vi "BRig_FPGA_v3,95.vi"() -> ()   [LabVIEW 2014]
uses:
  <vilib>/rvi/Emulation/niFpgaGetClockAttributes.vi
  <vilib>/rvi/Emulation/niFpgaSctlEmulationGetInTimedLoop.vi
  <vilib>/rvi/Emulation/niFpgaEmulationReportErrorSimple.vi
  <vilib>/rvi/eio/common/nirviEmuTemplateMethod_errors.vi
  <vilib>/rvi/Emulation/niFpgaCriticalErrorInLSC.vi
  <vilib>/eio/EIONode/EIONode.xnode
panel:
  out "AnaIn_1_0":u16
  out "AnaIn_1_1":u16
  out "AnaIn_1_2":u16
  out "AnaIn_1_3":u16
  out "AnaIn_1_4":u16
  out "AnaIn_0_4":u16
  out "AnaIn_0_3":u16
  out "AnaIn_0_2":u16
  out "AnaIn_0_1":u16
  out "AnaIn_0_0":u16
  in  "AI_newCycleFlag":bool
  in  "AnaOut1_Pair":u16
  in  "AnaOut0_Pair":u16
  out "fpga_solenoid_R":bool
  out "fpga_solenoid_L":bool
  out "fpga_laser2":bool
  out "fpga_laser1":bool
  in  "L2Led_ON":bool
  in  "L1Led_ON":bool
  in  "Rising(F)_or_Falling(T)":bool
  in  "Solenoid_trig_R":bool
  in  "Solenoid_trig_L":bool
  in  "Solenoid_nTotal_R":u32=100
  in  "Solenoid_nTotal_L":u32=100
  in  "L2Led_Baseline":bool
  in  "L1Led_Baseline":bool
  in  "CueLed_Baseline":bool
  in  "I_allReward":bool
  in  "AnaOut_1":u16
  in  "CueLed_Event":bool
  in  "CueLed_nValley":u32=100
  in  "CueLed_nPeak":u32=100
  in  "LC_Event_l2":bool
  in  "LC_Laser_l2":bool
  in  "LC_nShutter_l2":u32=100
  in  "LC_nValley_l2":u32=100
  in  "LC_nPeak_l2":u32=100
  in  "LR_wrong_nDelay_l2":u32
  in  "LR_reward_nDelay_l2":u32
  in  "LR_wrong_nTotal_l2":u32=100
  in  "LR_reward_nTotal_l2":u32=100
  in  "LR_wrong_laser_l2":bool
  in  "LR_wrong_Event_l2":bool
  in  "LR_reward_Laser_l2":bool
  in  "LR_reward_Event_l2":bool
  out "AnaIn_1":u16
  out "AnaIn_0":u16
  out "timeTrial_count":u32
  in  "timeTrial_trig":bool
  in  "k1__counter_per_ms":u16=100 min=100 max=40000 step=1
  in  "LC_nShutter_l1":u32=100
  in  "AnaOut_0":u16
  in  "LC_nValley_l1":u32=100
  in  "LC_nPeak_l1":u32=100
  in  "LC_Event_l1":bool
  in  "LR_wrong_nTotal_l1":u32=100
  in  "LR_wrong_nDelay_l1":u32
  in  "LR_reward_nTotal_l1":u32=100
  in  "LR_reward_nDelay_l1":u32
  in  "LR_reward_Event_l1":bool
  in  "LR_wrong_Event_l1":bool
  out "SelectWrong":bool
  out "SelectReward":bool
  in  "LR_wrong_Laser_l1":bool
  in  "LR_reward_Laser_l1":bool
  in  "Left(F)_or_Right(T)":bool
  in  "ignoreWrong":bool
  in  "SelectionState":bool
  in  "LC_Laser_l1":bool
  in  "FPGA_Stop":bool
  in  "audioTrigger_L":bool
  in  "audioTrigger_R":bool
  in  "audioFreq_L_kHz":u8=14 min=1 max=14 step=1
  in  "audioAmp_L":u16=1 min=1 max=32767 step=1
  in  "audioFreq_R_kHz":u8=14 min=1 max=14 step=1
  in  "audioAmp_R":u16=1 min=1 max=32767 step=1
  in  "A3_SL":bool
  in  "A1_SR":bool
  in  "Counts_Reset":bool
  out "A4_LickR":u32
  out "A2_LickL":u32
  in  "A6_Act":bool
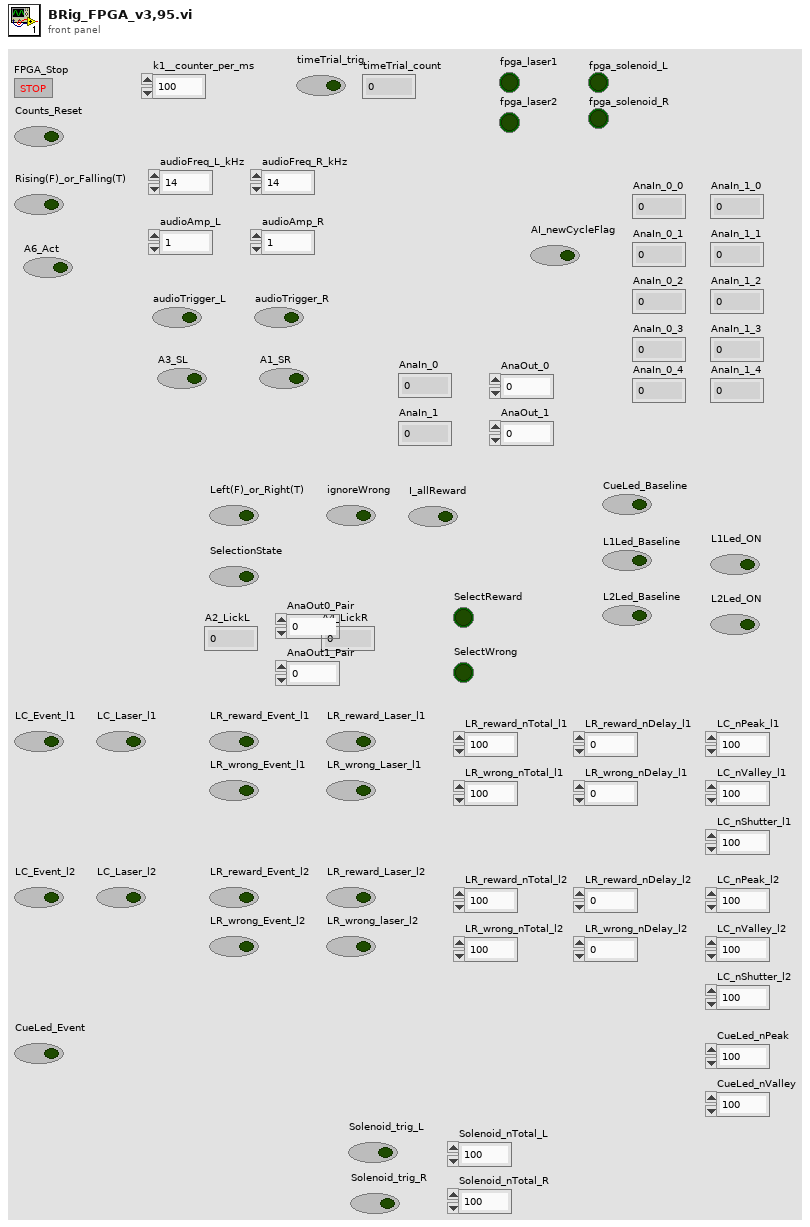
[diagram p1: front panel]
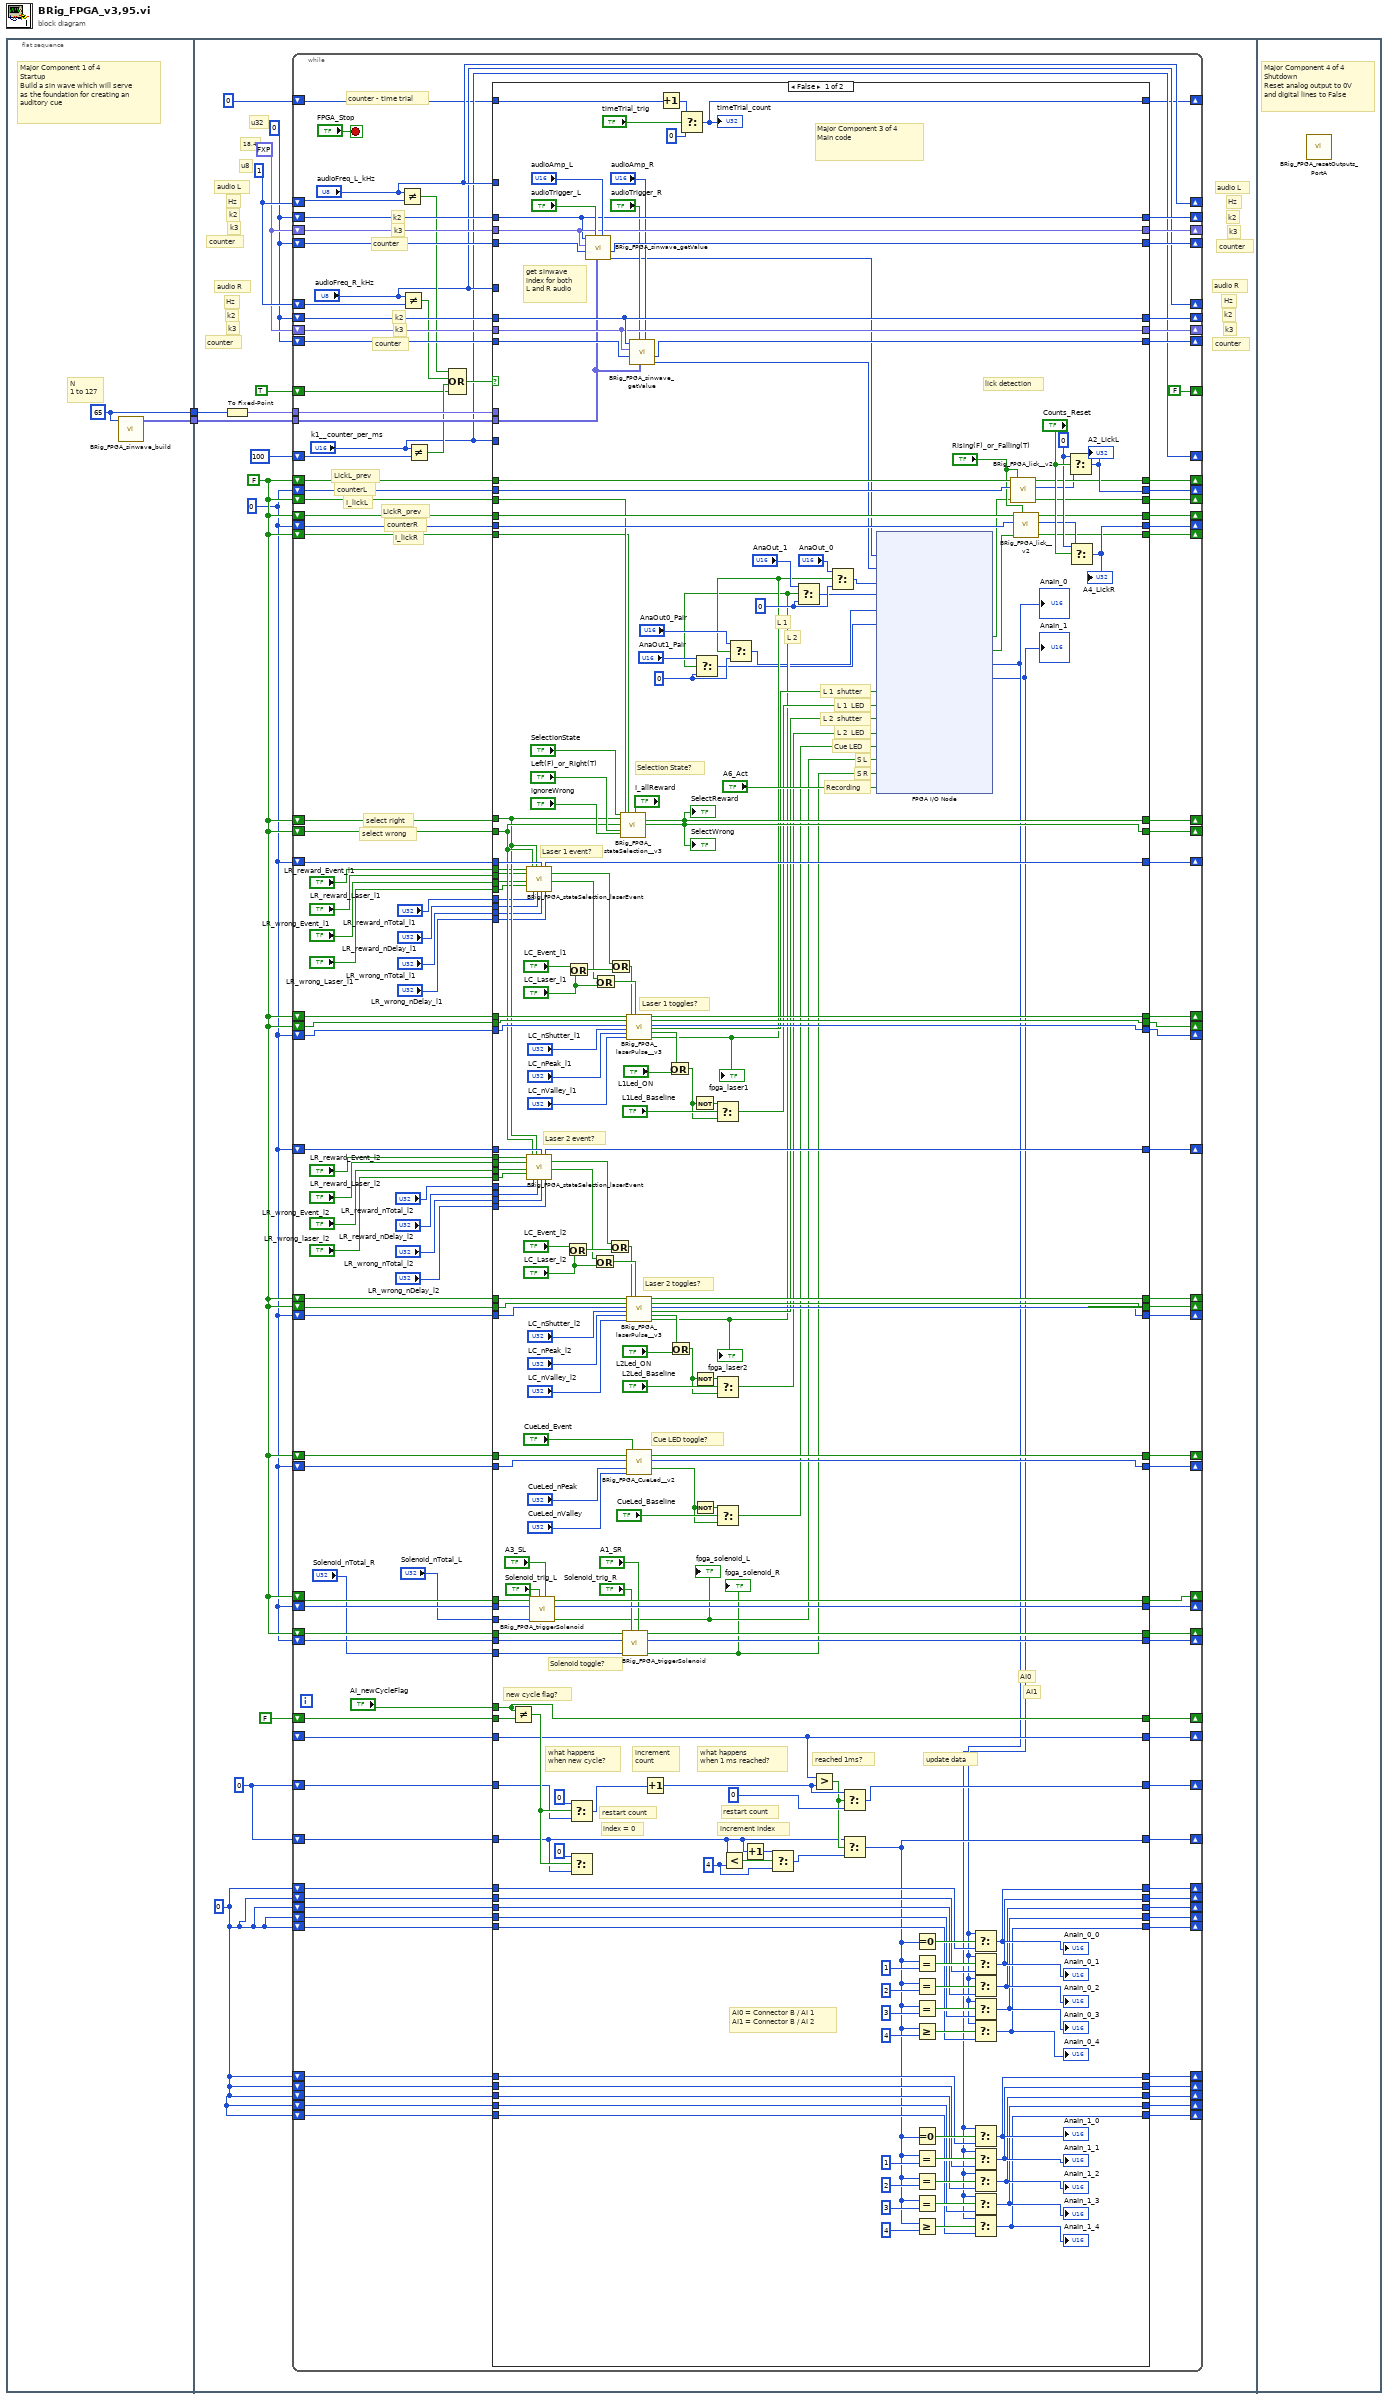
[diagram p0: block diagram]
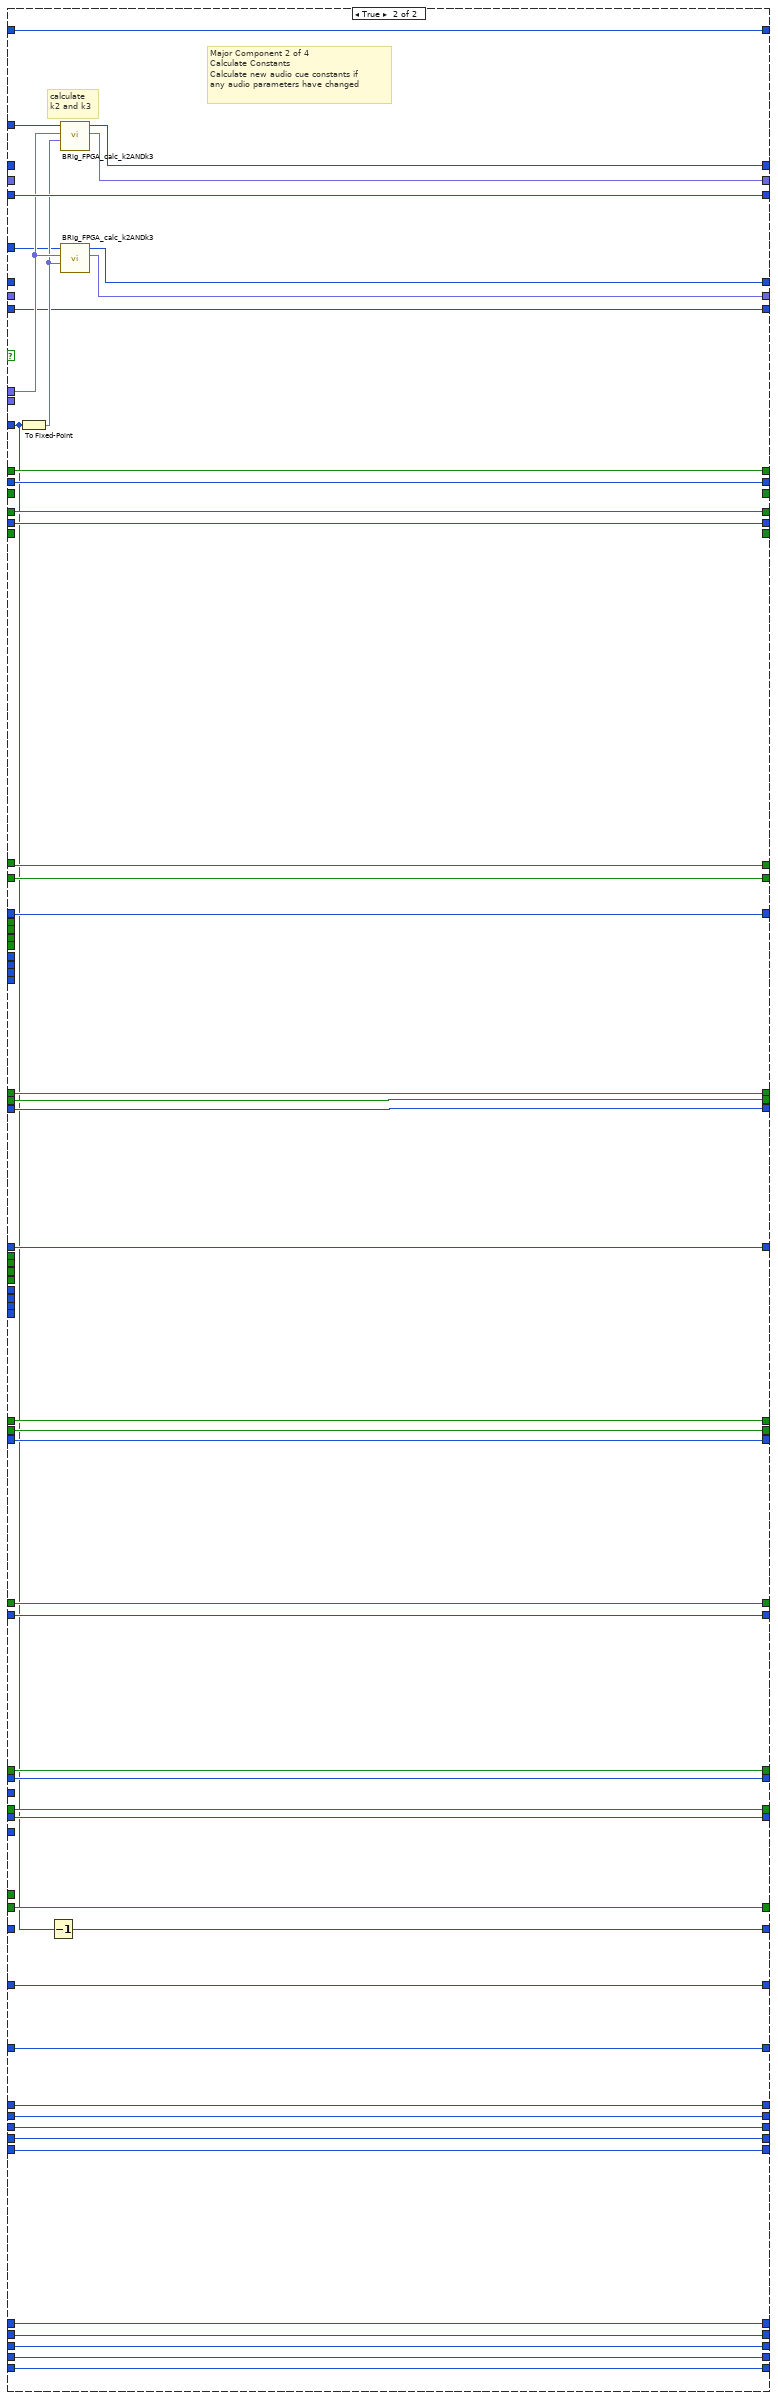
[diagram p2: hidden frame]
diagram:
  n1 = flat-sequence {
    tunnel: [w4] -> w2
    tunnel: [w3] -> w1
    tunnel: w2 -> [w18]
    tunnel: w1 -> [w17]
    frame #0 {
      w3 = 65 ("dimension size")
      # "Major Component 1 of 4\nStartup\nBuild a sin wave which will serve\nas the foundation for creating an\nauditory cue"
      # "N\n1 to 127"
      n2 = call "BRig_FPGA_sinwave_build.vi"("input_Npts"=w3) -> ("output_array_sin"=w4:fxp<+/-,16,2>[])  [unwired: 10 in]
    }
    frame #1 {
      w6 = u16 0
      w5 = u16 0
      w8 = u32 0
      w9 = FALSE
      w13 = u32 0
      w14 = fxp<+,18,4> 0.0
      w15 = u8 1
      # "counter"
      # "k3"
      # "k2"
      # "counter"
      # "k3"
      # "k2"
      # "counter"
      # "counter"
      # "u32"
      # "k3"
      # "k2"
      # "k3"
      # "18,4"
      # "u8"
      # "Hz"
      # "Hz"
      # "audio R"
      # "audio L"
      # "Hz"
      # "k2"
      # "Hz"
      # "audio R"
      # "audio L"
      n3 = To Fixed-Point(number=w17) -> (fixed-point=w16:fxp<+,7,7>)  [unwired: 1 in]
      n4 = while {
        shift-right: ["audioFreq_L_kHz"] -> _
        shift-left: w15 -> [w138]
        shift-right: [w132] -> _
        shift-left: w13 -> [w136]
        shift-right: ["audioFreq_R_kHz"] -> _
        shift-left: w15 -> [w128]
        tunnel: w18 -> [w135]
        tunnel: w16 -> [w134]
        shift-right: [w131] -> _
        shift-left: w14 -> [w133]
        shift-right: [w129] -> _
        shift-left: w13 -> [w130]
        shift-right: [w126] -> _
        shift-left: w13 -> [w127]
        shift-right: [w124] -> _
        shift-left: w14 -> [w125]
        shift-right: [w122] -> _
        shift-left: w13 -> [w123]
        shift-right: ["k1__counter_per_ms"] -> _
        shift-left: u16 100 ("y") -> [w121]
        shift-right: [FALSE] -> _
        shift-left: TRUE -> [w116]
        shift-right: [w109] -> _
        shift-left: w9 -> [w111]
        shift-right: [w108] -> _
        shift-left: w9 -> [w110]
        shift-right: [w106] -> _
        shift-left: w8 -> [w107]
        shift-right: [w104] -> _
        shift-left: w8 -> [w105]
        shift-right: [w101] -> _
        shift-left: w9 -> [w103]
        shift-right: [w100] -> _
        shift-left: w9 -> [w102]
        shift-right: [w98] -> _
        shift-left: w9 -> [w99]
        shift-right: [w96] -> _
        shift-left: w9 -> [w97]
        shift-right: [w94] -> _
        shift-left: u32 0 -> [w95]
        shift-right: [w92] -> _
        shift-left: w8 -> [w93]
        shift-right: [w91] -> _
        shift-left: w9 -> [w88]
        shift-right: [w90] -> _
        shift-left: w9 -> [w87]
        shift-right: [w89] -> _
        shift-left: w8 -> [w86]
        shift-right: [w84] -> _
        shift-left: w8 -> [w85]
        shift-right: [w83] -> _
        shift-left: w9 -> [w80]
        shift-right: [w82] -> _
        shift-left: w9 -> [w79]
        shift-right: [w81] -> _
        shift-left: w8 -> [w78]
        shift-right: [w77] -> _
        shift-left: w9 -> [w75]
        shift-right: [w76] -> _
        shift-left: w8 -> [w74]
        shift-right: [w56] -> _
        shift-left: w8 -> [w57]
        shift-right: [w53] -> _
        shift-left: w9 -> [w55]
        shift-right: [w50] -> _
        shift-left: w9 -> [w52]
        shift-right: [w49] -> _
        shift-left: w8 -> [w51]
        shift-right: [w33] -> _
        shift-left: FALSE -> [w46]
        shift-right: [w32] -> _
        shift-left: w6 -> [w44]
        shift-right: [w31] -> _
        shift-left: w6 -> [w43]
        shift-right: [w30] -> _
        shift-left: w5 -> [w45]
        shift-right: [w29] -> _
        shift-left: w5 -> [w41]
        shift-right: [w28] -> _
        shift-left: w5 -> [w40]
        shift-right: [w27] -> _
        shift-left: w5 -> [w39]
        shift-right: [w26] -> _
        shift-left: w5 -> [w42]
        shift-right: [w25] -> _
        shift-left: w5 -> [w38]
        shift-right: [w24] -> _
        shift-left: w5 -> [w37]
        shift-right: [w23] -> _
        shift-left: w5 -> [w36]
        shift-right: [w22] -> _
        shift-left: w5 -> [w35]
        shift-right: [w21] -> _
        shift-left: w5 -> [w34]
        shift-right: [w20] -> _
        shift-left: _ -> [w19]
        stop <- "FPGA_Stop" stop-if-true
        # "counter"
        # "k3"
        # "k2"
        # "counter"
        # "k3"
        # "k2"
        # "counter - time trial"
        # "I_lickR"
        # "counterR"
        # "LickR_prev"
        # "I_lickL"
        # "counterL"
        # "LickL_prev"
        # "select wrong"
        # "select right"
        n5 = Not Equal?(x="audioFreq_L_kHz", y=w138) -> (x != y?=w120:bool)
        n6 = Not Equal?(x="audioFreq_R_kHz", y=w128) -> (x != y?=w119:bool)
        n7 = Not Equal?(x="k1__counter_per_ms", y=w121) -> (x != y?=w117:bool)
        n8 = Compound Arithmetic op=OR(w120, w119, w117, w116) -> (w118:bool)
        n9 = case shown="False" w118 {
          tunnel: w136 -> [w334 _]
          tunnel: "audioFreq_L_kHz" -> [_ w395]
          tunnel: w135 -> [w327 _]
          tunnel: w134 -> [_ w391]
          tunnel: "k1__counter_per_ms" -> [_ w352]
          tunnel: w133 -> [w335 _]
          tunnel: [w334 w394] -> w132
          tunnel: [w335 w393] -> w131
          tunnel: w130 -> [w339 w392]
          tunnel: [w336 w392] -> w129
          tunnel: w127 -> [w331 _]
          tunnel: [w331 w387] -> w126
          tunnel: w125 -> [w330 _]
          tunnel: [w330 w388] -> w124
          tunnel: w123 -> [w333 w386]
          tunnel: "audioFreq_R_kHz" -> [_ w389]
          tunnel: [w332 w386] -> w122
          tunnel: w111 -> [w322 w385]
          tunnel: w110 -> [w321 w384]
          tunnel: [w326 w385] -> w109
          tunnel: [w319 w384] -> w108
          tunnel: w107 -> [w323 w383]
          tunnel: [w349 w383] -> w106
          tunnel: w105 -> [w320 w382]
          tunnel: [w346 w382] -> w104
          tunnel: w103 -> [w277 w381]
          tunnel: w102 -> [w278 w380]
          tunnel: [w297 w381] -> w101
          tunnel: [w342 w380] -> w100
          tunnel: [w312 w377] -> w91
          tunnel: [w313 w376] -> w90
          tunnel: [w314 w375] -> w89
          tunnel: w99 -> [w316 _]
          tunnel: [w325 _] -> w98
          tunnel: w97 -> [w315 _]
          tunnel: [w317 _] -> w96
          tunnel: w95 -> [w304 w379]
          tunnel: [w301 w379] -> w94
          tunnel: w93 -> [w296 w378]
          tunnel: [w295 w378] -> w92
          tunnel: w88 -> [w294 w377]
          tunnel: w87 -> [w293 w376]
          tunnel: w86 -> [w292 w375]
          tunnel: w85 -> [w280 w374]
          tunnel: [w279 w374] -> w84
          tunnel: [w275 w373] -> w83
          tunnel: [w274 w372] -> w82
          tunnel: [w273 w371] -> w81
          tunnel: w80 -> [w272 w373]
          tunnel: w79 -> [w271 w372]
          tunnel: w78 -> [w270 w371]
          tunnel: [w267 w370] -> w77
          tunnel: [w266 w369] -> w76
          tunnel: w75 -> [w265 w370]
          tunnel: w74 -> [w264 w369]
          tunnel: "LR_reward_Event_l1" -> [w250 _]
          tunnel: "LR_reward_Laser_l1" -> [w249 _]
          tunnel: "LR_wrong_Event_l1" -> [w248 _]
          tunnel: "LR_wrong_Laser_l1" -> [w247 _]
          tunnel: "LR_reward_nTotal_l1" -> [w246 _]
          tunnel: "LR_reward_nDelay_l1" -> [w245 _]
          tunnel: "LR_wrong_nTotal_l1" -> [w244 _]
          tunnel: "LR_wrong_nDelay_l1" -> [w243 _]
          tunnel: "LR_reward_Event_l2" -> [w242 _]
          tunnel: "LR_reward_Laser_l2" -> [w241 _]
          tunnel: "LR_wrong_Event_l2" -> [w240 _]
          tunnel: "LR_wrong_laser_l2" -> [w239 _]
          tunnel: "LR_reward_nTotal_l2" -> [w238 _]
          tunnel: "LR_reward_nDelay_l2" -> [w237 _]
          tunnel: "LR_wrong_nTotal_l2" -> [w236 _]
          tunnel: "LR_wrong_nDelay_l2" -> [w235 _]
          tunnel: w57 -> [w234 w368]
          tunnel: [w229 w368] -> w56
          tunnel: w55 -> [w233 w367]
          tunnel: "Solenoid_nTotal_L" -> [w232 _]
          tunnel: [w228 w367] -> w53
          tunnel: w52 -> [w225 w366]
          tunnel: w51 -> [w224 w365]
          tunnel: [w223 w366] -> w50
          tunnel: [w222 w365] -> w49
          tunnel: "Solenoid_nTotal_R" -> [w221 _]
          tunnel: "AI_newCycleFlag" -> [w154 _]
          tunnel: w46 -> [w167 w364]
          tunnel: w45 -> [w166 w362]
          tunnel: w44 -> [w165 w351]
          tunnel: w43 -> [w164 w363]
          tunnel: w42 -> [w163 w358]
          tunnel: w41 -> [w162 w361]
          tunnel: w40 -> [w161 w360]
          tunnel: w39 -> [w160 w359]
          tunnel: w38 -> [w159 w357]
          tunnel: w37 -> [w158 w356]
          tunnel: w36 -> [w157 w355]
          tunnel: w35 -> [w156 w354]
          tunnel: w34 -> [w155 w353]
          tunnel: [w154 w364] -> w33
          tunnel: [w152 w351] -> w32
          tunnel: [w151 w363] -> w31
          tunnel: [w148 w362] -> w30
          tunnel: [w147 w361] -> w29
          tunnel: [w146 w360] -> w28
          tunnel: [w145 w359] -> w27
          tunnel: [w144 w358] -> w26
          tunnel: [w143 w357] -> w25
          tunnel: [w142 w356] -> w24
          tunnel: [w141 w355] -> w23
          tunnel: [w140 w354] -> w22
          tunnel: [w139 w353] -> w21
          tunnel: w19 -> [w153 _]
          tunnel: [w153 w350] -> w20
          frame False {
            w186 = u16 4 ("y")
            w202 = u16 0 ("f")
            w261 = u16 0 ("f")
            w347 = u32 0 ("t")
            # "AI0 = Connector B / AI 1\nAI1 = Connector B / AI 2"
            # "increment index"
            # "restart count"
            # "index = 0"
            # "restart count"
            # "AI1"
            # "AI0"
            # "update data"
            # "reached 1ms?"
            # "increment\ncount"
            # "what happens\nwhen new cycle?"
            # "what happens\nwhen 1 ms reached?"
            # "new cycle flag?"
            # "Cue LED"
            # "L 2  shutter"
            # "L 2  LED"
            # "L 1  shutter"
            # "L 1  LED"
            # "Recording"
            # "S L"
            # "S R"
            # "L 2"
            # "L 1"
            # "Solenoid toggle?"
            # "Cue LED toggle?"
            # "Laser 2 toggles?"
            # "Laser 2 event?"
            # "Laser 1 toggles?"
            # "Selection State?"
            # "Laser 1 event?"
            # "Major Component 3 of 4\nMain code"
            # "get sinwave\nindex for both\nL and R audio"
            # "lick detection"
            n10 = Not Equal?(x=w154, y=w167) -> (x != y?=w192:bool)
            n11 = call "BRig_FPGA_stateSelection_laserEvent.vi"("I_LR_reward"=w250, "I_LR_reward_laser"=w249, "I_LR_wrong"=w248, "I_LR_wrong_laser"=w247, "I_selectWrong"=w278, "laser_reward_nTotal"=w246, "I_selectReward"=w277, "laser_reward_nDelay"=w245, "counter"=w296, "laser_wrong_nTotal"=w244, "laser_wrong_nDelay"=w243) -> ("output_counter"=w295:u32, "output_I_laserEvent"=w291:bool, "output_I_laserOn"=w290:bool)  [unwired: 6 in]
            n12 = call "BRig_FPGA_stateSelection_laserEvent.vi"("I_LR_reward"=w242, "I_LR_reward_laser"=w241, "I_LR_wrong"=w240, "I_LR_wrong_laser"=w239, "I_selectWrong"=w278, "laser_reward_nTotal"=w238, "I_selectReward"=w277, "laser_reward_nDelay"=w237, "counter"=w280, "laser_wrong_nTotal"=w236, "laser_wrong_nDelay"=w235) -> ("output_counter"=w279:u32, "output_I_laserEvent"=w276:bool, "output_I_laserOn"=w281:bool)  [unwired: 6 in]
            n13 = call "BRig_FPGA_triggerSolenoid.vi"("input_Solenoid_MTrig"="A3_SL", "input_Solenoid_trig"="Solenoid_trig_L", "input_threshold"=w232, "input_counter"=w234, "input_trig"=w233) -> ("output_Solenoid_OnOff"=w205:bool, "output_counter"=w229:u32, "output_trig"=w228:bool)  [unwired: 4 in]
            "fpga_solenoid_L" <- w205
            n14 = Or(x="LC_Event_l2", y="LC_Laser_l2") -> (x .or. y?=w285:bool)
            n15 = Or(x="LC_Event_l1", y="LC_Laser_l1") -> (x .or. y?=w308:bool)
            n16 = Select(t=u16 0, s=w192, f=w165) -> (s? t:f=w191:u16)
            n17 = Select(t=u16 0 ("f"), s=w192, f=w164) -> ()  [unwired: 1 out]
            n18 = call "BRig_FPGA_sinwave_getValue.vi"("audioAmp"="audioAmp_L", "sinwave"=w327, "audioTrigger"="audioTrigger_L", "counter"=w339, "k3"=w335, "k2"=w334) -> ("output_audioValue"=w299:i16, "output_counter"=w336:u32)  [unwired: 4 in]
            n19 = Or(x=w281, y="LC_Laser_l2") -> (x .or. y?=w283:bool)
            n20 = Or(x=w290, y="LC_Laser_l1") -> (x .or. y?=w306:bool)
            n21 = Or(x=w276, y=w285) -> (x .or. y?=w282:bool)
            n22 = Or(x=w291, y=w308) -> (x .or. y?=w305:bool)
            n23 = call "BRig_FPGA_stateSelection__v3.vi"("I_selectionState"="SelectionState", "I_selectRight"=w277, "I_selectWrong"=w278, "I_Left(F)_or_Right(T)"="Left(F)_or_Right(T)", "I_ignoreWrong"="ignoreWrong", "I_lickL"=w316, "I_lickR"=w315, "I_allReward"="I_allReward") -> ("output__I_selectRight"=w297:bool, "output__I_selectWrong"=w342:bool)  [unwired: 18 in]
            "SelectWrong" <- w342
            "SelectReward" <- w297
            n24 = call "BRig_FPGA_triggerSolenoid.vi"("input_Solenoid_MTrig"="A1_SR", "input_Solenoid_trig"="Solenoid_trig_R", "input_threshold"=w221, "input_counter"=w224, "input_trig"=w225) -> ("output_Solenoid_OnOff"=w204:bool, "output_counter"=w222:u32, "output_trig"=w223:bool)  [unwired: 4 in]
            "fpga_solenoid_R" <- w204
            n25 = call "BRig_FPGA_laserPulse__v3.vi"("I_shutter"=w294, "I_peak"=w293, "count"=w292, "laser_Nshutter"="LC_nShutter_l1", "laser_Npeak"="LC_nPeak_l1", "laser_Nvalley"="LC_nValley_l1", "I_laserEvent"=w305, "I_laser"=w306) -> ("output_I_shutter"=w312:bool, "output_I_peak"=w313:bool, "output_count"=w314:u32, "output_shutter"=w210:bool, "output_led"=w218:bool, "output_laser"=w200:bool)  [unwired: 6 in]
            "fpga_laser1" <- w200
            n26 = call "BRig_FPGA_laserPulse__v3.vi"("I_shutter"=w272, "I_peak"=w271, "count"=w270, "laser_Nshutter"="LC_nShutter_l2", "laser_Npeak"="LC_nPeak_l2", "laser_Nvalley"="LC_nValley_l2", "I_laserEvent"=w282, "I_laser"=w283) -> ("output_I_shutter"=w275:bool, "output_I_peak"=w274:bool, "output_count"=w273:u32, "output_shutter"=w208:bool, "output_led"=w215:bool, "output_laser"=w199:bool)  [unwired: 6 in]
            "fpga_laser2" <- w199
            n27 = call "BRig_FPGA_CueLed__v2.vi"("I_peak"=w265, "count"=w264, "laser_Npeak"="CueLed_nPeak", "laser_Nvalley"="CueLed_nValley", "I_CueLed_Event"="CueLed_Event") -> ("output_I_peak"=w267:bool, "output_count"=w266:u32, "output_led"=w255:bool)  [unwired: 12 in]
            n28 = call "BRig_FPGA_sinwave_getValue.vi"("audioAmp"="audioAmp_R", "sinwave"=w327, "audioTrigger"="audioTrigger_R", "counter"=w333, "k3"=w330, "k2"=w331) -> ("output_audioValue"=w298:i16, "output_counter"=w332:u32)  [unwired: 4 in]
            n29 = Increment(x=w191) -> (x+1=w190:u16)
            n30 = Increment(x=w304) -> (x+1=w303:u32)
            n31 = Or(x=w218, y="L1Led_ON") -> (x .or. y?=w217:bool)
            n32 = Or(x=w215, y="L2Led_ON") -> (x .or. y?=w214:bool)
            n33 = Select(t=w303, s="timeTrial_trig", f=u32 0) -> (s? t:f=w301:u32)
            "timeTrial_count" <- w301
            n34 = Not(x=w217) -> (.not. x?=w254:bool)
            n35 = Not(x=w214) -> (.not. x?=w252:bool)
            n36 = Not(x=w255) -> (.not. x?=w257:bool)
            n37 = Select(t="AnaOut1_Pair", s=w199, f=w202) -> (s? t:f=w198:u16)
            n38 = Select(t=w254, s="L1Led_Baseline", f=w217) -> (s? t:f=w209:bool)
            n39 = Select(t=w252, s="L2Led_Baseline", f=w214) -> (s? t:f=w207:bool)
            n40 = Select(t=w257, s="CueLed_Baseline", f=w255) -> (s? t:f=w206:bool)
            n41 = Less?(x=w164, y=w186) -> (x < y?=w196:bool)
            n42 = Select(t="AnaOut0_Pair", s=w200, f=w202) -> (s? t:f=w197:u16)
            n43 = Increment(x=w164) -> (x+1=w195:u16)
            n44 = Select(t=w195, s=w196, f=w186) -> (s? t:f=w187:u16)
            n45 = Select(t="AnaOut_1", s=w199, f=w261) -> (s? t:f=w259:u16)
            n46 = Greater?(x=w153, y=w190) -> (0:w188:bool)
            n47 = Select(t="AnaOut_0", s=w200, f=w261) -> (s? t:f=w262:u16)
            n48 = Select(t=w190, s=w188, f=u16 0) -> (s? t:f=w152:u16)
            n49 = Select(t=w164, s=w188, f=w187) -> (s? t:f=w151:u16)
            n50 = xnode "FPGA I/O Node"("AudioOut/Left"=w299, "AudioOut/Right"=w298, "ConnectorB/AO0"=w262, "ConnectorB/AO1"=w259, "ConnectorA/AO0"=w197, "ConnectorA/AO1"=w198, "ConnectorA/DIO6"=w210, "ConnectorB/DIO14"=w209, "ConnectorA/DIO7"=w208, "ConnectorB/DIO15"=w207, "ConnectorB/DIO9"=w206, "ConnectorA/DIO3"=w205, "ConnectorA/DIO5"=w204, "ConnectorA/DIO0"="A6_Act") -> ("ConnectorA/DIO4"=w213:bool, "ConnectorA/DIO2"=w212:bool, "ConnectorB/AI1"=w150:u16, "ConnectorB/AI2"=w149:u16)  [unwired: 18 in, 18 out]
            "AnaIn_0" <- w150
            "AnaIn_1" <- w149
            n51 = Equal To 0?(x=w151) -> (x = 0?=w185:bool)
            n52 = Equal?(x=w151, y=u16 1) -> (x = y?=w180:bool)
            n53 = Equal?(x=w151, y=u16 2) -> (x = y?=w179:bool)
            n54 = Equal?(x=w151, y=u16 3) -> (x = y?=w178:bool)
            n55 = Greater Or Equal?(x=w151, y=u16 4) -> (x >= y?=w177:bool)
            n56 = Equal To 0?(x=w151) -> (x = 0?=w168:bool)
            n57 = Equal?(x=w151, y=u16 1) -> (x = y?=w173:bool)
            n58 = Equal?(x=w151, y=u16 2) -> (x = y?=w174:bool)
            n59 = Equal?(x=w151, y=u16 3) -> (x = y?=w175:bool)
            n60 = Greater Or Equal?(x=w151, y=u16 4) -> (x >= y?=w176:bool)
            n61 = Select(t=w150, s=w185, f=w166) -> (s? t:f=w148:u16)
            "AnaIn_0_0" <- w148
            n62 = Select(t=w150, s=w180, f=w162) -> (s? t:f=w147:u16)
            "AnaIn_0_1" <- w147
            n63 = Select(t=w150, s=w179, f=w161) -> (s? t:f=w146:u16)
            "AnaIn_0_2" <- w146
            n64 = Select(t=w150, s=w178, f=w160) -> (s? t:f=w145:u16)
            "AnaIn_0_3" <- w145
            n65 = Select(t=w150, s=w177, f=w163) -> (s? t:f=w144:u16)
            "AnaIn_0_4" <- w144
            n66 = Select(t=w149, s=w168, f=w159) -> (s? t:f=w143:u16)
            "AnaIn_1_0" <- w143
            n67 = Select(t=w149, s=w173, f=w158) -> (s? t:f=w142:u16)
            "AnaIn_1_1" <- w142
            n68 = Select(t=w149, s=w174, f=w157) -> (s? t:f=w141:u16)
            "AnaIn_1_2" <- w141
            n69 = Select(t=w149, s=w175, f=w156) -> (s? t:f=w140:u16)
            "AnaIn_1_3" <- w140
            n70 = Select(t=w149, s=w176, f=w155) -> (s? t:f=w139:u16)
            "AnaIn_1_4" <- w139
            n71 = call "BRig_FPGA_lick__v2.vi"("Rising(F)_or_Falling(T)"="Rising(F)_or_Falling(T)", "I_stateDetector_new"=w213, "counter"=w323, "I_stateDetector_prev"=w322) -> ("output_I_lick"=w325:bool, "output_counter"=w324:u32, "output_I_stateDetector_prev"=w326:bool)  [unwired: 5 in]
            n72 = call "BRig_FPGA_lick__v2.vi"("Rising(F)_or_Falling(T)"="Rising(F)_or_Falling(T)", "I_stateDetector_new"=w212, "counter"=w320, "I_stateDetector_prev"=w321) -> ("output_I_lick"=w317:bool, "output_counter"=w318:u32, "output_I_stateDetector_prev"=w319:bool)  [unwired: 5 in]
            n73 = Select(t=w347, s="Counts_Reset", f=w324) -> (s? t:f=w349:u32)
            "A2_LickL" <- w349
            n74 = Select(t=w347, s="Counts_Reset", f=w318) -> (s? t:f=w346:u32)
            "A4_LickR" <- w346
          }
          frame True {
            # "Major Component 2 of 4\nCalculate Constants\nCalculate new audio cue constants if\nany audio parameters have changed"
            # "calculate\nk2 and k3"
            n75 = To Fixed-Point(number=w352) -> (fixed-point=w390:fxp<+,16,16>)  [unwired: 1 in]
            n76 = Decrement(x=w352) -> (x-1=w350:u16)
            n77 = call "BRig_FPGA_calc_k2ANDk3.vi"("input_k1[count/ms]"=w390, "input_Npts"=w391, "input_freq[kHz]"=w395) -> ("output_k3"=w393:fxp<+,18,4>, "output_k2"=w394:u32)  [unwired: 7 in]
            n78 = call "BRig_FPGA_calc_k2ANDk3.vi"("input_k1[count/ms]"=w390, "input_Npts"=w391, "input_freq[kHz]"=w389) -> ("output_k3"=w388:fxp<+,18,4>, "output_k2"=w387:u32)  [unwired: 7 in]
          }
        }
      }
    }
    frame #2 {
      # "Major Component 4 of 4\nShutdown\nReset analog output to 0V\nand digital lines to False"
      n79 = call "BRig_FPGA_resetOutputs_PortA.vi"() -> ()  [unwired: 12 in]
    }
  }
